vi "main.vi"() -> ()   [LabVIEW 2017]
uses:
  <vilib>/printing/ReportDocExtensions.llb/Append Front Panel Image to Report (path).vi
  <vilib>/Utility/NIReport.llb/NI_report.lvclass
  <vilib>/Utility/NIReport.llb/NI_ReportGenerationCore.lvlib
panel:
  out "T[C/K]":dbl(slide) scale=0.0..100.0
  out "?":dbl(graph)
  in  "?":bool
  out "Alarm":bool
  in  "[C/K]":bool
  in  "Crit temp [C]":dbl
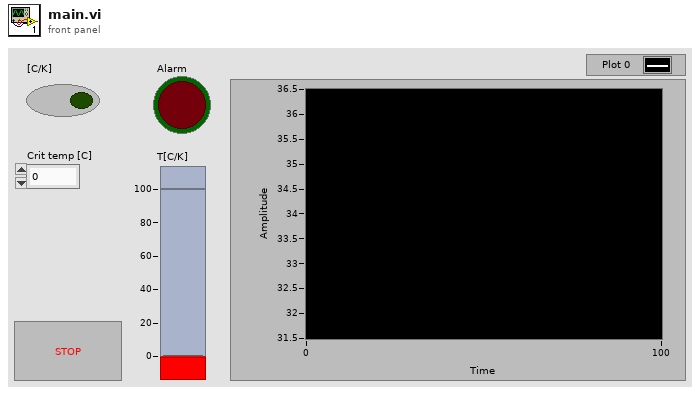
[diagram p1: front panel]
types:
  T1 = enum16{"Standard Report", "HTML", "Word", "Excel"}
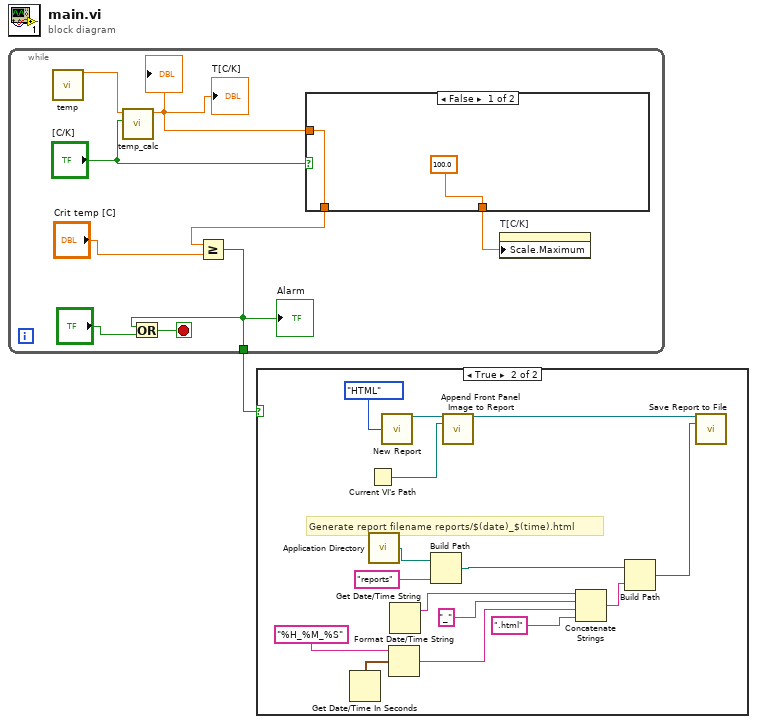
[diagram p0: block diagram]
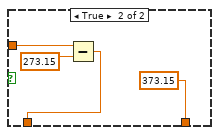
[diagram p3: hidden frame]
diagram:
  n1 = while {
    tunnel: [w6] -> w1
    stop <- w9 stop-if-true
    n2 = call "temp.vi"() -> ("T (F)"=w10:dbl)  [unwired: 15 in]
    n3 = call "temp_calc.vi"("[C/K]"="[C/K]", "T (F)"=w10) -> ("Out temp [C/K]"=w3:dbl)  [unwired: 9 in]
    "?" <- w3
    "T[C/K]" <- w3
    n4 = case shown="False" "[C/K]" {
      tunnel: w3 -> [w12 w16]
      tunnel: [w12 w14] -> w4
      tunnel: [100.0 ("Scale.Range:Maximum") 373.15 ("Scale.Range:Maximum")] -> w2
      frame False {
      }
      frame True {
        n5 = Subtract(x=w16, y=273.15) -> (x-y=w14:dbl)
      }
    }
    n6 = Greater Or Equal?(x=w4, y="Crit temp [C]") -> (x >= y?=w6:bool)
    "Alarm" <- w6
    n7 = Or(x=w6, y="?") -> (x .or. y?=w9:bool)
    n8 = property on="T[C/K]" class="Slide (strict)"("Scale.Maximum"=w2) -> ()  [unwired: 2 in, 2 out]
  }
  n9 = case shown="True" w1 {
    frame False {
    }
    frame True {
      # "Generate report filename reports/$(date)_$(time).html"
      n10 = Get Date/Time In Seconds() -> (seconds since 1Jan1904=w19:timestamp)
      n11 = Current VI's Path() -> (path=w26:path)
      n12 = call <vilib>:"Application Directory.vi"() -> ("Application Directory"=w28:path)
      n13 = call <vilib>:"New Report.vi"("report type"=T1."HTML") -> ("report out"=w30:refnum<class "NI_report.lvclass">)  [unwired: 13 in, 1 out]
      n14 = Format Date/Time String(time format string (%c)="%H_%M_%S", seconds (now)=w19) -> (date/time string=w17:string)  [unwired: 1 in]
      n15 = Get Date/Time String() -> (date string=w25:string)  [unwired: 3 in, 1 out]
      n16 = Build Path(base path=w28, name or relative path="reports") -> (appended path=w22:path)
      n17 = call-poly <vilib>:"Append Front Panel Image to Report.vi"("report in"=w30, "VI"=w26) -> ("report out"=w29:refnum<class "NI_report.lvclass">)  [unwired: 9 in, 4 out]
      n18 = Concatenate Strings(w25, "_" ("string"), w17, ".html" ("string")) -> (w21:string)
      n19 = Build Path(base path=w22, name or relative path=w21) -> (appended path=w20:path)
      n20 = call-dynamic "Save Report to File.vi"("report in"=w29, "report file path"=w20) -> ()  [unwired: 12 in, 2 out]
    }
  }
